vi "Close.vi"(8 "Error In":errorcluster, 11 "object in":refnum<class "Scope Base.lvclass">) -> (0 "Error Out":errorcluster, 3 "object out":refnum<class "Scope Base.lvclass">)   [LabVIEW 2023, in "Scope.lvlib" / "Scope Base.lvlib" / "Scope Base.lvclass"]
uses:
  Scope Base.lvclass
  Scope Base.lvclass/Scope Base.ctl
  Interfaces/IConfigure/IConfigure.lvclass
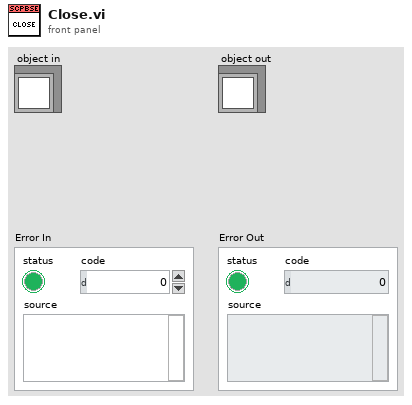
[diagram p1: front panel]
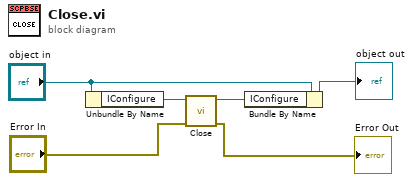
[diagram p0: block diagram]
diagram:
  n1 = Unbundle By Name("object in") -> ("IConfigure"=w5:refnum<class "IConfigure.lvclass">)
  n2 = call-dynamic "Close.vi"("error in"="Error In", "IConfigure in"=w5) -> ("error out"=→"Error Out":errorcluster, "IConfigure out"=w1:refnum<class "IConfigure.lvclass">)  [unwired: 8 in]
  n3 = Bundle By Name(cluster="object in", "IConfigure"=w1) -> (→"object out":refnum<class "Scope Base.lvclass">)
